vi "DeletingIndex.vi"(8 "error in (no error)":errorcluster, 9 "New":u32[](array[numeric]), 10 "Old":u32[](array[numeric]), 11 "Input":dbl[][](array[numeric])=[[nan, 1.0, nan, nan, nan, 5.0, 6.0, nan, nan, nan, 10.0], [nan, nan, nan, nan, nan, nan, nan, nan, nan, nan, nan], [nan, nan, nan, nan, nan, nan, nan, nan, nan, nan, nan], [nan, nan, nan, nan, nan, nan, nan, nan, nan, nan, nan], [nan, nan, nan, nan, nan, nan, nan, nan, nan, nan, nan], [nan, nan, nan, nan, nan, nan, nan, nan, nan, nan, nan], [nan, nan, nan, nan, nan, nan, nan, nan, nan, nan, nan], [nan, nan, nan, nan, nan, nan, nan, nan, nan, nan, nan], [nan, nan, nan, nan, nan, nan, nan, nan, nan, nan, nan], [nan, nan, nan, nan, nan, nan, nan, nan, nan, nan, nan]]) -> (0 "error out":errorcluster, 3 "Output":dbl[][](array[numeric]))   [LabVIEW 2015]
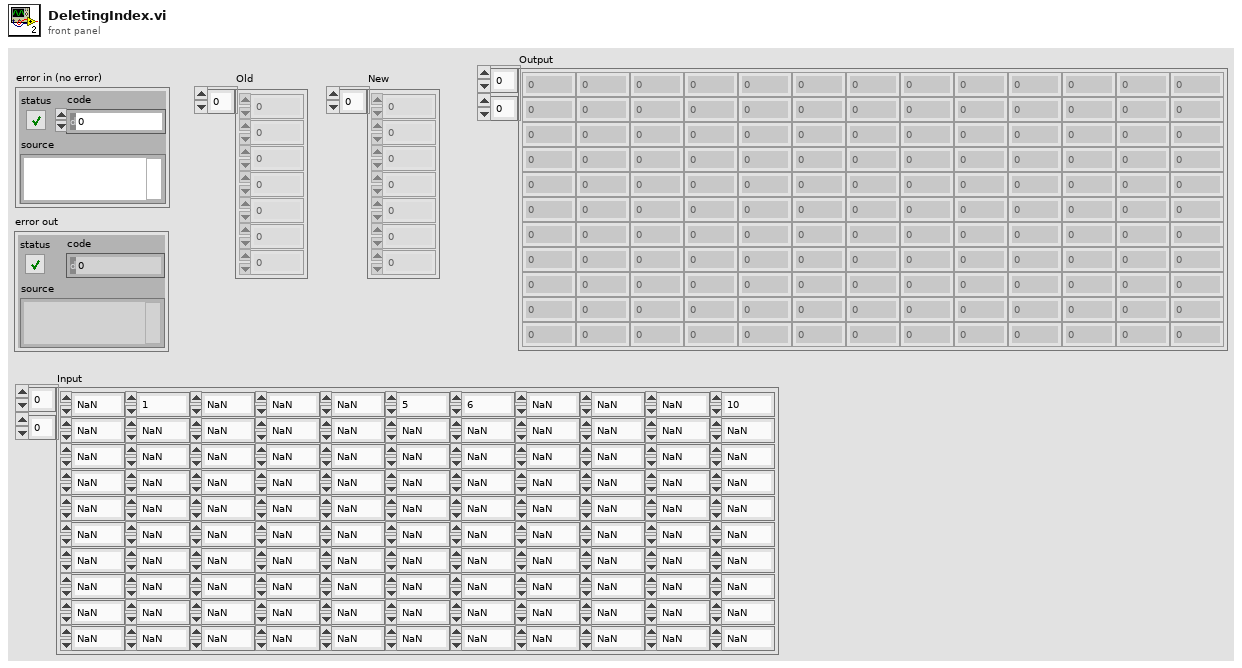
[diagram p1: front panel]
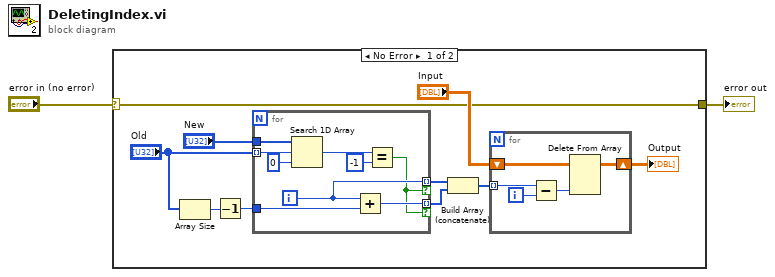
[diagram p0: block diagram]
diagram:
  n1 = case shown="No Error" "error in (no error)" {
    selector: "error in (no error)" -> [w3 w27]
    tunnel: [w3 w27] -> w1
    frame No Error {
      n2 = Array Size(array="Old") -> (size(s)=w10:i32)
      n3 = Decrement(x=w10) -> (x-1=w9:i32)
      n4 = for {
        tunnel: "New" -> [w25]
        tunnel: "Old" -> [w24] mode=indexing
        tunnel: [w20] -> w8 mode=indexing if=w18
        tunnel: w9 -> [w21]
        tunnel: [w19] -> w7 mode=indexing if=w18
        i -> [w20]
        n5 = Search 1D Array(1D array=w25, element=w24, start index (0)=0) -> (index of element=w26:i32)
        n6 = Add(x=w20, y=w21) -> (x+y=w19:i32)
        n7 = Equal?(x=w26, y=-1) -> (x = y?=w18:bool)
      }
      n8 = Build Array (concatenate)(w8, w7) -> (w5:i32[])
      n9 = for {
        tunnel: w5 -> [w14] mode=indexing
        shift-right: [w16] -> w4
        shift-left: "Input" -> [w17]
        i -> [w13]
        n10 = Subtract(x=w14, y=w13) -> (x-y=w15:i32)
        n11 = Delete From Array(array=w17, index (col)=w15) -> (array with subset deleted=w16:dbl[][])  [unwired: 2 in, 1 out]
      }
      "Output" <- w4
    }
    frame Error {
    }
  }
  "error out" <- w1
